vi "sub_logdata.vi"(8 "error in":errorcluster, 10 "data_str":string, 11 "Title":string) -> (0 "ERROR OUT":errorcluster caption="error out")   [LabVIEW 2018]
uses:
  Global_val.vi
panel:
  out "Path out":path
  out "dup path":path
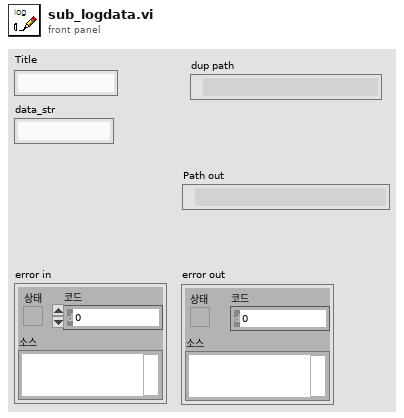
[diagram p1: front panel]
types:
  T1 = enum16{"open", "replace", "create", "open or create", "replace or create", "replace or create with confirmation"}
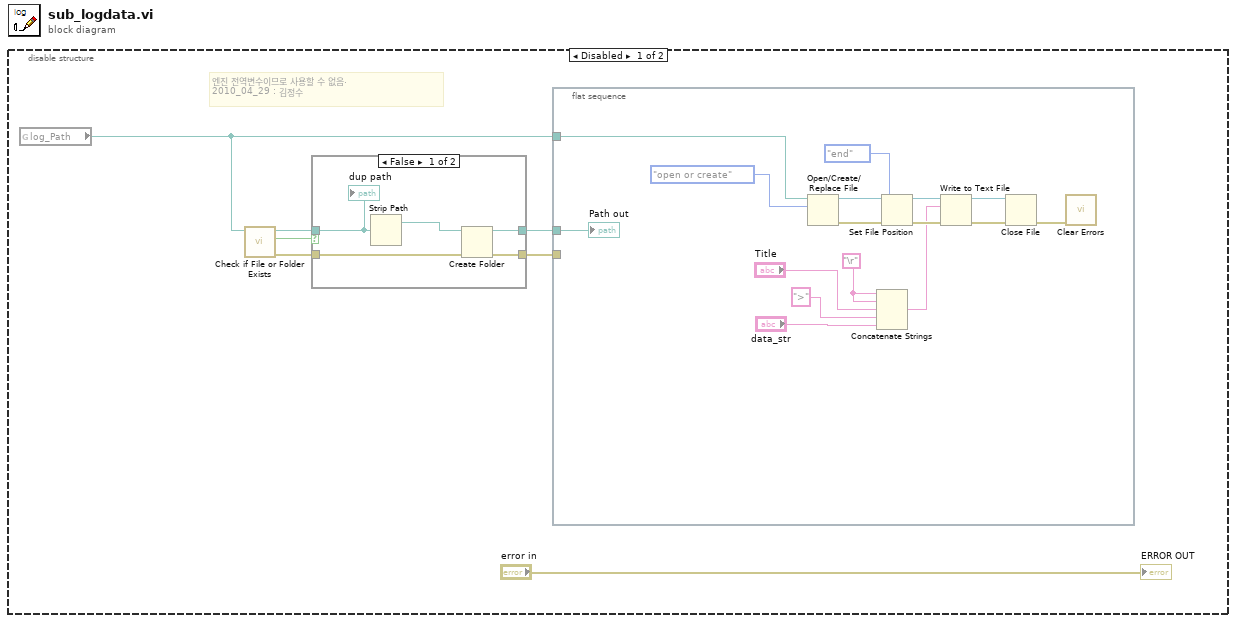
[diagram p0: block diagram]
diagram:
  n1 = disable-structure shown="Disabled" {
    frame Disabled {
      # "엔진 전역변수이므로 사용할 수 없음.\n2010_04_29 : 김정수"
      n2 = global read "Global_val.vi" "log_Path"() -> (w1:path)
      n3 = call <vilib>:"Check if File or Folder Exists.vi"("path"=w1) -> ("error out"=w5:errorcluster, "file or folder exists?"=w7:bool, "dup path"=w6:path)  [unwired: 8 in]
      n4 = case shown="False" w7 {
        tunnel: w6 -> [w26 w30]
        tunnel: w5 -> [w28 w29]
        tunnel: [w27 w30] -> w4
        tunnel: [w24 w29] -> w3
        frame False {
          n5 = Strip Path(path=w26) -> (stripped path=w25:path)  [unwired: 1 out]
          n6 = Create Folder(path (use dialog)=w25, error in=w28) -> (created path=w27:path, error out=w24:errorcluster)  [unwired: 1 in, 1 out]
          "dup path" <- w26
        }
        frame True {
        }
      }
      n7 = flat-sequence {
        tunnel: w4 -> [w23]
        tunnel: w1 -> [w22]
        tunnel: w3 -> [_]
        frame #0 {
          w8 = "\r"
          n8 = Open/Create/Replace File(file path (use dialog)=w22, operation (0:open)=T1."open or create" ("동작(0:open)")) -> (refnum out=w14:refnum<file>, error out=w15:errorcluster)  [unwired: 4 in, 1 out]
          n9 = Concatenate Strings(w8, w8, "Title", ">" ("문자열"), "data_str") -> (w11:string)
          n10 = Set File Position(refnum=w14, from (0:start)=enum16{"start", "end", "current"}."end" ("시작(0:시작)"), error in=w15) -> (refnum out=w13:refnum<file>, error out=w12:errorcluster)  [unwired: 1 in]
          n11 = Write to Text File(file (use dialog)=w13, text=w11, error in=w12) -> (refnum out=w17:refnum<file>, error out=w18:errorcluster)  [unwired: 1 in, 1 out]
          n12 = Close File(refnum=w17, error in=w18) -> (error out=w9:errorcluster)  [unwired: 1 out]
          n13 = call <vilib>:"Clear Errors.vi"("error in (no error)"=w9) -> ()  [unwired: 5 in, 2 out]
          "Path out" <- w23
        }
      }
      "ERROR OUT" <- "error in"
    }
    frame Enabled {
    }
  }
